vi "rs3_ReadDepthPreference3.vi"(0 "file (use dialog)":path) -> (1 "HDAD 2*":T1={"lambdaCensus"=126.0, "lambdaAD"=800.0, "ignoreSAD"=0}, 3 "ST Color Control 2":T4, 4 "depth control 2":T8={"plusIncrement (47)"=19, "MinusDecrement (46)"=4, "deepSeaMedianThreshold (48)"=554, "scoreThreshA(49)"=1, "scoreThreshB (50)"=632, "textureDifferenceThreshold (52)"=0, "textureCountThreshold (51)"=32, "deepSea2ndPeakThresh.(53)"=665, "deepSeaNeighborThresh.(54)"=126, "IrAgreeThreshold (55)"=11}, 6 "ST RSM 2":T7={"rsmBypass (56)"=0, "diffThresh (57)"=6.49, "sloRauDiffThresh(58)"=0.305, "removeThresh(59)"=60}, 9 "text":string="{\n    \"param-disableraucolor\": 0,\n    \"param-disablesadcolor\": 0,\n    \"param-disablesadnormalize\": 0,\n    \"param-disablesloleftcolor\": 0,\n    \"param-disableslorightcolor\": 0,\n    \"param-lambdaad\": 833,\n    \"param-lambdacensus\": 26,\n    \"param-leftrightthreshold\": 11,\n    \"param-maxscorethreshb\": 632,\n    \"param-medianthreshold\": 554,\n    \"param-minscorethresha\": 1,\n    \"param-neighborthresh\": 126,\n    \"param-raumine\": 7,\n    \"param-rauminn\": 1,\n    \"param-rauminnssum\": 7,\n    \"param-raumins\": 3,\n    \"param-rauminw\": 5,\n    \"param-rauminwesum\": 12,\n    \"param-regioncolorthresholdb\": 0.26379450841061053,\n    \"param-regioncolorthresholdg\": 0.9806201235330119,\n    \"param-regioncolorthresholdr\": 0.013826660558426103,\n    \"param-regionshrinku\": 4,\n    \"param-regionshrinkv\": 1,\n    \"param-regionspatialthresholdu\": 7,\n    \"param-regionspatialthresholdv\": 3,\n    \"param-robbinsmonrodecrement\": 4,\n    \"param-robbinsmonroincrement\": 19,\n    \"param-rsmdiffthreshold\": 1.0367311077984247,\n    \"param-rsmrauslodiffthreshold\": 0.8955340364089305,\n    \"param-rsmremovethreshold\": 0.7604262237190709,\n    \"param-scanlineedgetaub\": 105,\n    \"param-scanlineedgetaug\": 442,\n    \"param-scanlineedgetaur\": 46,\n    \"param-scanlinep1\": 93,\n    \"param-scanlinep1onediscon\": 70,\n    \"param-scanlinep1twodiscon\": 92,\n    \"param-scanlinep2\": 473,\n    \"param-scanlinep2onediscon\": 123,\n    \"param-scanlinep2twodiscon\": 409,\n    \"param-secondpeakdelta\": 665,\n    \"param-texturecountthresh\": 32,\n    \"param-texturedifferencethresh\": 0,\n    \"param-usersm\": 1\n}", 10 "ST SLO Penalty 2":T6={"sloK1Penalty (79)"=10, "sloK2Penalty (80)"=60, "sloK1PenaltyMod1(81)"=84, "sloK2PenaltyMod1(82)"=56, "sloK1PenaltyMod2(83)"=59, "sloK2PenaltyMod2(84)"=4}, 12 "ST SLO Threshold 2":T2={"SLOdiffThreshRed(76)"=200, "SLODiffThreshGreen(77)"=200, "SLODiffThreshBlue(78)"=200}, 13 "error out":errorcluster, 14 "ST Rau Threshold 2":T3={"rauDiffThreshRed(73)"=70, "rauDiffThreshGreen(74)"=70, "rauDiffThreshBlue(75)"=70}, 15 "ST RAU vector 2":T5={"minWest (60)"=7, "minEast (61)"=7, "minWEsum (62)"=12, "minNorth (63)"=3, "minSouth (64)"=2, "minNSSum(65)"=1, "uStrink (66)"=2, "vShrink (67)"=1})   [LabVIEW 2019, in "libRealSense3.lvlib"]
uses:
  libRealSense3.lvlib
panel:
  in  "error in (no error)":errorcluster
  # "RS2 Read Depth Preferences"
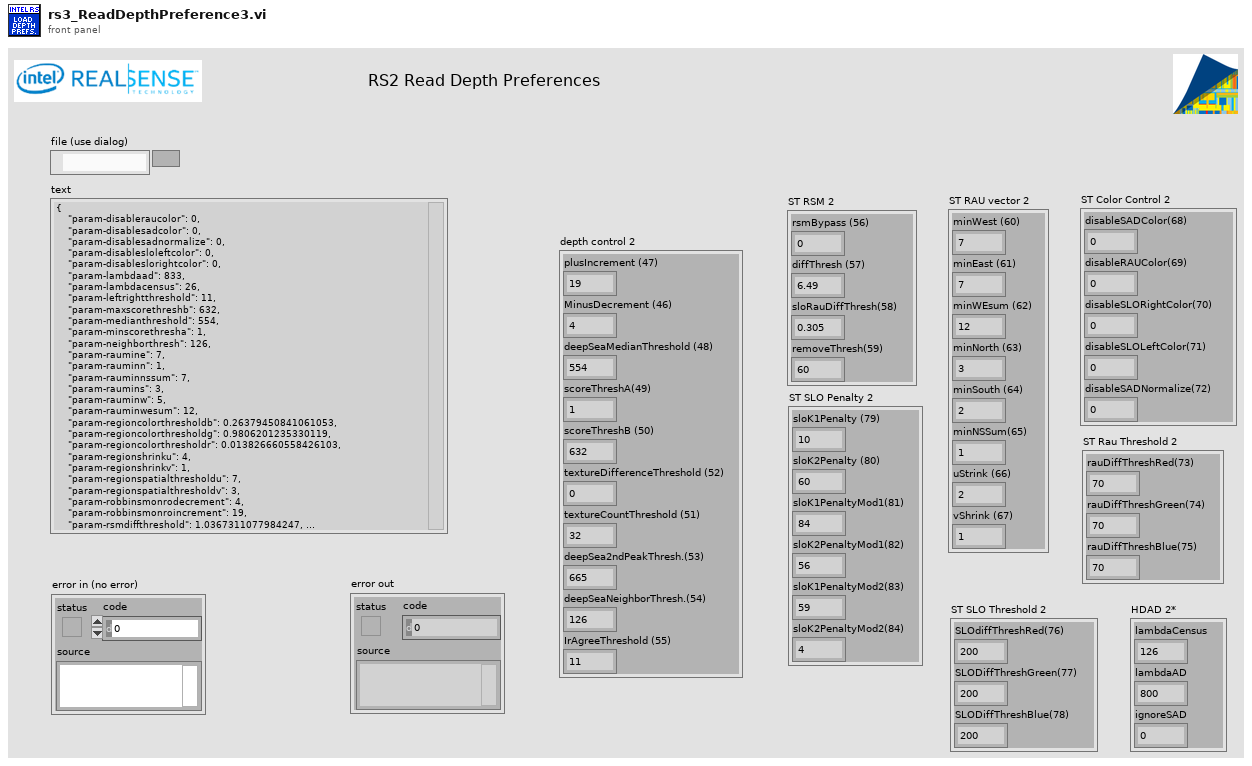
[diagram p1: front panel]
types:
  T1 = cluster{"lambdaCensus":sgl, "lambdaAD":sgl, "ignoreSAD":u32}
  T2 = cluster{"SLOdiffThreshRed(76)":u32, "SLODiffThreshGreen(77)":u32, "SLODiffThreshBlue(78)":u32}
  T3 = cluster{"rauDiffThreshRed(73)":u32, "rauDiffThreshGreen(74)":u32, "rauDiffThreshBlue(75)":u32}
  T4 = cluster{"disableSADColor(68)":u32, "disableRAUColor(69)":u32, "disableSLORightColor(70)":u32, "disableSLOLeftColor(71)":u32, "disableSADNormalize(72)":u32}
  T5 = cluster{"minWest (60)":u32, "minEast (61)":u32, "minWEsum (62)":u32, "minNorth (63)":u32, "minSouth (64)":u32, "minNSSum(65)":u32, "uStrink (66)":u32, "vShrink (67)":u32}
  T6 = cluster{"sloK1Penalty (79)":u32, "sloK2Penalty (80)":u32, "sloK1PenaltyMod1(81)":u32, "sloK2PenaltyMod1(82)":u32, "sloK1PenaltyMod2(83)":u32, "sloK2PenaltyMod2(84)":u32}
  T7 = cluster{"rsmBypass (56)":u32, "diffThresh (57)":sgl, "sloRauDiffThresh(58)":sgl, "removeThresh(59)":u32}
  T8 = cluster{"plusIncrement (47)":u32, "MinusDecrement (46)":u32, "deepSeaMedianThreshold (48)":u32, "scoreThreshA(49)":u32, "scoreThreshB (50)":u32, "textureDifferenceThreshold (52)":u32, "textureCountThreshold (51)":u32, "deepSea2ndPeakThresh.(53)":u32, "deepSeaNeighborThresh.(54)":u32, "IrAgreeThreshold (55)":u32}
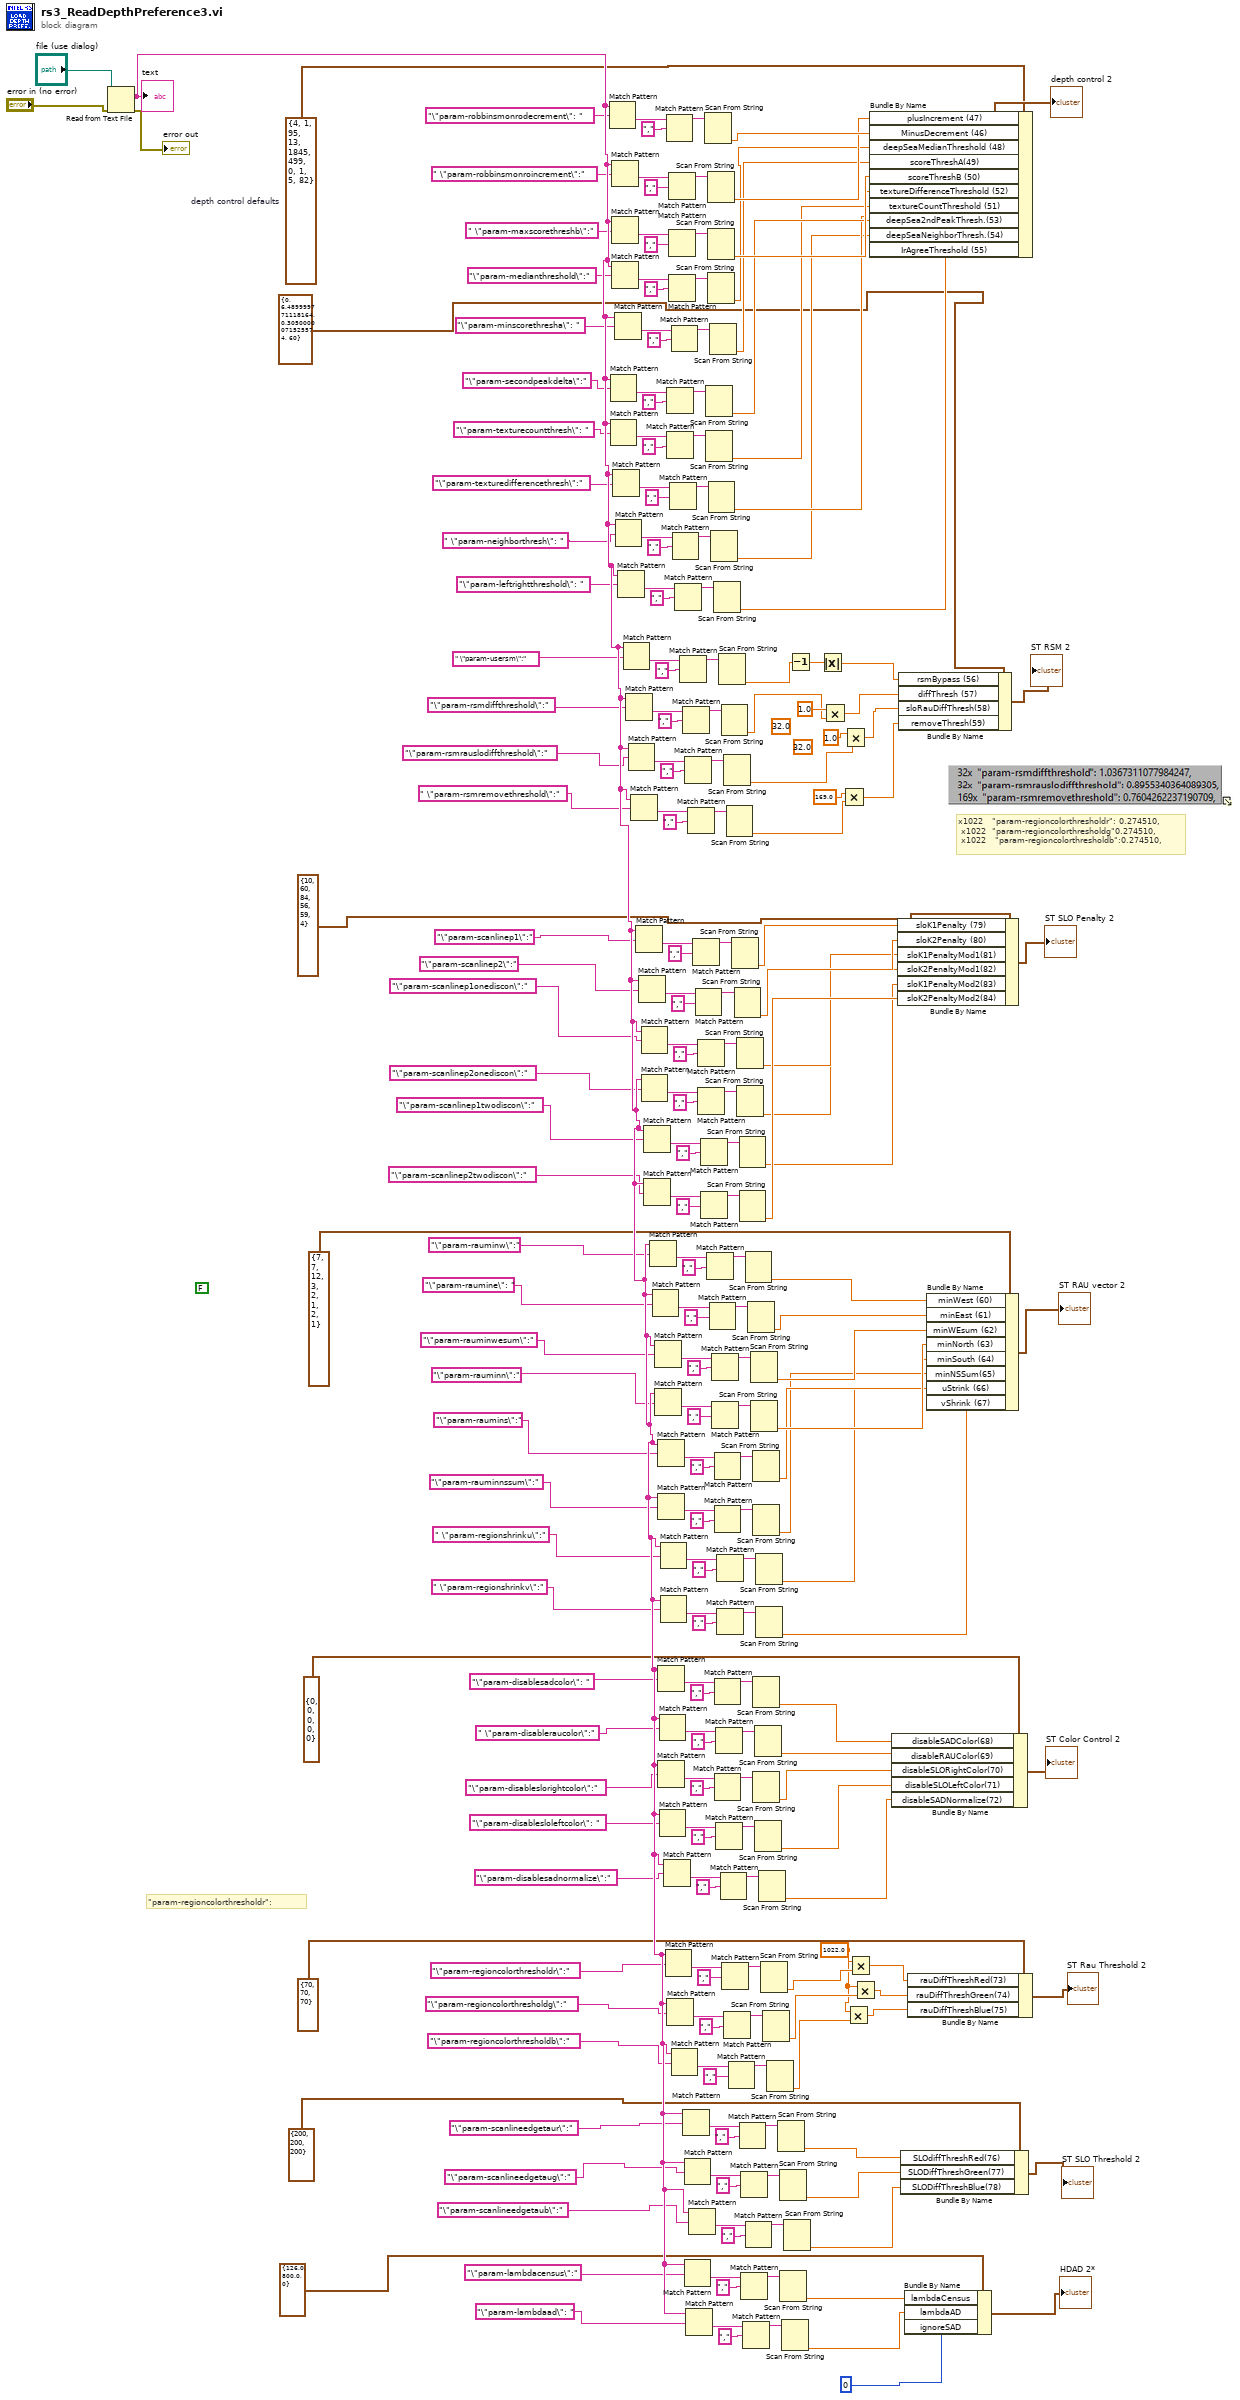
[diagram p0: block diagram]
diagram:
  (unwired) 32.0 ("x")
  (unwired) 32.0 ("x")
  w8 = 1022.0
  w229 = T8 {"plusIncrement (47)"=4, "MinusDecrement (46)"=1, "deepSeaMedianThreshold (48)"=95, "scoreThreshA(49)"=13, "scoreThreshB (50)"=1845, "textureDifferenceThreshold (52)"=499, "textureCountThreshold (51)"=0, "deepSea2ndPeakThresh.(53)"=1, "deepSeaNeighborThresh.(54)"=5, "IrAgreeThreshold (55)"=82}  # depth control defaults
  (unwired) FALSE
  # "x1022   \"param-regioncolorthresholdr\": 0.274510, \n x1022  \"param-regioncolorthresholdg\"0.274510, \n x1022   \"param-regioncolorthresholdb\":0.274510,"
  # "\"param-regioncolorthresholdr\":"
  n1 = Read from Text File(file (use dialog)="file (use dialog)", error in="error in (no error)") -> (text=w238:string, error out=→"error out":errorcluster)  [unwired: 2 in, 2 out]
  "text" <- w238
  n2 = Match Pattern(string=w238, regular expression="\"param-robbinsmonrodecrement\": ") -> (after substring=w235:string)  [unwired: 1 in, 3 out]
  n3 = Match Pattern(string=w238, regular expression="\"param-secondpeakdelta\":") -> (after substring=w203:string)  [unwired: 1 in, 3 out]
  n4 = Match Pattern(string=w238, regular expression="\"param-texturecountthresh\": ") -> (after substring=w208:string)  [unwired: 1 in, 3 out]
  n5 = Match Pattern(string=w238, regular expression=" \"param-robbinsmonroincrement\":") -> (after substring=w232:string)  [unwired: 1 in, 3 out]
  n6 = Match Pattern(string=w238, regular expression=" \"param-maxscorethreshb\":") -> (after substring=w224:string)  [unwired: 1 in, 3 out]
  n7 = Match Pattern(string=w238, regular expression="\"param-medianthreshold\":") -> (after substring=w219:string)  [unwired: 1 in, 3 out]
  n8 = Match Pattern(string=w238, regular expression="\"param-texturedifferencethresh\":") -> (after substring=w209:string)  [unwired: 1 in, 3 out]
  n9 = Match Pattern(string=w238, regular expression="\"param-minscorethresha\": ") -> (after substring=w218:string)  [unwired: 1 in, 3 out]
  n10 = Match Pattern(string=w238, regular expression=" \"param-neighborthresh\": ") -> (after substring=w194:string)  [unwired: 1 in, 3 out]
  n11 = Match Pattern(string=w238, regular expression="\"param-leftrightthreshold\": ") -> (after substring=w193:string)  [unwired: 1 in, 3 out]
  n12 = Match Pattern(string=w238, regular expression=" \"param-usersm\":") -> (after substring=w175:string)  [unwired: 1 in, 3 out]
  n13 = Match Pattern(string=w238, regular expression="\"param-rsmdiffthreshold\":") -> (after substring=w174:string)  [unwired: 1 in, 3 out]
  n14 = Match Pattern(string=w238, regular expression="\"param-rsmrauslodiffthreshold\":") -> (after substring=w180:string)  [unwired: 1 in, 3 out]
  n15 = Match Pattern(string=w238, regular expression=" \"param-rsmremovethreshold\":") -> (after substring=w181:string)  [unwired: 1 in, 3 out]
  n16 = Match Pattern(string=w238, regular expression="\"param-scanlinep1\":") -> (after substring=w162:string)  [unwired: 1 in, 3 out]
  n17 = Match Pattern(string=w238, regular expression="\"param-scanlinep2\":") -> (after substring=w159:string)  [unwired: 1 in, 3 out]
  n18 = Match Pattern(string=w238, regular expression="\"param-scanlinep1onediscon\":") -> (after substring=w158:string)  [unwired: 1 in, 3 out]
  n19 = Match Pattern(string=w238, regular expression="\"param-scanlinep2onediscon\":") -> (after substring=w153:string)  [unwired: 1 in, 3 out]
  n20 = Match Pattern(string=w238, regular expression="\"param-scanlinep1twodiscon\":") -> (after substring=w152:string)  [unwired: 1 in, 3 out]
  n21 = Match Pattern(string=w238, regular expression="\"param-scanlinep2twodiscon\":") -> (after substring=w143:string)  [unwired: 1 in, 3 out]
  n22 = Match Pattern(string=w238, regular expression="\"param-rauminw\":") -> (after substring=w115:string)  [unwired: 1 in, 3 out]
  n23 = Match Pattern(string=w238, regular expression="\"param-raumine\": ") -> (after substring=w118:string)  [unwired: 1 in, 3 out]
  n24 = Match Pattern(string=w238, regular expression="\"param-rauminwesum\":") -> (after substring=w119:string)  [unwired: 1 in, 3 out]
  n25 = Match Pattern(string=w238, regular expression="\"param-rauminn\":") -> (after substring=w124:string)  [unwired: 1 in, 3 out]
  n26 = Match Pattern(string=w238, regular expression="\"param-raumins\":") -> (after substring=w125:string)  [unwired: 1 in, 3 out]
  n27 = Match Pattern(string=w238, regular expression="\"param-rauminnssum\":") -> (after substring=w130:string)  [unwired: 1 in, 3 out]
  n28 = Match Pattern(string=w238, regular expression="\"param-disablesadcolor\": ") -> (after substring=w88:string)  [unwired: 1 in, 3 out]
  n29 = Match Pattern(string=w238, regular expression="\"param-disableslorightcolor\":") -> (after substring=w77:string)  [unwired: 1 in, 3 out]
  n30 = Match Pattern(string=w238, regular expression=" \"param-disableraucolor\":") -> (after substring=w83:string)  [unwired: 1 in, 3 out]
  n31 = Match Pattern(string=w238, regular expression="\"param-disablesloleftcolor\": ") -> (after substring=w82:string)  [unwired: 1 in, 3 out]
  n32 = Match Pattern(string=w238, regular expression=" \"param-regionshrinku\":") -> (after substring=w112:string)  [unwired: 1 in, 3 out]
  n33 = Match Pattern(string=w238, regular expression=" \"param-regionshrinkv\":") -> (after substring=w107:string)  [unwired: 1 in, 3 out]
  n34 = Match Pattern(string=w238, regular expression="\"param-disablesadnormalize\":") -> (after substring=w74:string)  [unwired: 1 in, 3 out]
  n35 = Match Pattern(string=w238, regular expression="\"param-regioncolorthresholdr\":") -> (after substring=w59:string)  [unwired: 1 in, 3 out]
  n36 = Match Pattern(string=w235, regular expression=",") -> (before substring=w237:string)  [unwired: 1 in, 3 out]
  n37 = Match Pattern(string=w203, regular expression=",") -> (before substring=w205:string)  [unwired: 1 in, 3 out]
  n38 = Match Pattern(string=w208, regular expression=",") -> (before substring=w206:string)  [unwired: 1 in, 3 out]
  n39 = Match Pattern(string=w238, regular expression="\"param-regioncolorthresholdg\":") -> (after substring=w54:string)  [unwired: 1 in, 3 out]
  n40 = Match Pattern(string=w232, regular expression=",") -> (before substring=w231:string)  [unwired: 1 in, 3 out]
  n41 = Match Pattern(string=w224, regular expression=",") -> (before substring=w222:string)  [unwired: 1 in, 3 out]
  n42 = Match Pattern(string=w219, regular expression=",") -> (before substring=w221:string)  [unwired: 1 in, 3 out]
  n43 = Match Pattern(string=w209, regular expression=",") -> (before substring=w211:string)  [unwired: 1 in, 3 out]
  n44 = Match Pattern(string=w218, regular expression=",") -> (before substring=w216:string)  [unwired: 1 in, 3 out]
  n45 = Match Pattern(string=w238, regular expression="\"param-regioncolorthresholdb\":") -> (after substring=w62:string)  [unwired: 1 in, 3 out]
  n46 = Match Pattern(string=w194, regular expression=",") -> (before substring=w196:string)  [unwired: 1 in, 3 out]
  n47 = Match Pattern(string=w193, regular expression=",") -> (before substring=w191:string)  [unwired: 1 in, 3 out]
  n48 = Match Pattern(string=w175, regular expression=",") -> (before substring=w177:string)  [unwired: 1 in, 3 out]
  n49 = Match Pattern(string=w174, regular expression=",") -> (before substring=w172:string)  [unwired: 1 in, 3 out]
  n50 = Match Pattern(string=w238, regular expression="\"param-scanlineedgetaur\":") -> (after substring=w45:string)  [unwired: 1 in, 3 out]
  n51 = Match Pattern(string=w238, regular expression="\"param-scanlineedgetaug\":") -> (after substring=w50:string)  [unwired: 1 in, 3 out]
  n52 = Match Pattern(string=w238, regular expression="\"param-lambdacensus\":") -> (after substring=w38:string)  [unwired: 1 in, 3 out]
  n53 = Match Pattern(string=w180, regular expression=",") -> (before substring=w178:string)  [unwired: 1 in, 3 out]
  n54 = Match Pattern(string=w238, regular expression="\"param-lambdaad\": ") -> (after substring=w33:string)  [unwired: 1 in, 3 out]
  n55 = Match Pattern(string=w181, regular expression=",") -> (before substring=w183:string)  [unwired: 1 in, 3 out]
  n56 = Match Pattern(string=w238, regular expression="\"param-scanlineedgetaub\":") -> (after substring=w42:string)  [unwired: 1 in, 3 out]
  n57 = Match Pattern(string=w162, regular expression=",") -> (before substring=w164:string)  [unwired: 1 in, 3 out]
  n58 = Match Pattern(string=w159, regular expression=",") -> (before substring=w161:string)  [unwired: 1 in, 3 out]
  n59 = Match Pattern(string=w158, regular expression=",") -> (before substring=w156:string)  [unwired: 1 in, 3 out]
  n60 = Match Pattern(string=w153, regular expression=",") -> (before substring=w155:string)  [unwired: 1 in, 3 out]
  n61 = Match Pattern(string=w152, regular expression=",") -> (before substring=w150:string)  [unwired: 1 in, 3 out]
  n62 = Match Pattern(string=w143, regular expression=",") -> (before substring=w145:string)  [unwired: 1 in, 3 out]
  n63 = Scan From String(input string=w237) -> (output 1=w228:dbl)  [unwired: 4 in, 3 out]
  n64 = Scan From String(input string=w205) -> (output 1=w199:dbl)  [unwired: 4 in, 3 out]
  n65 = Scan From String(input string=w206) -> (output 1=w198:dbl)  [unwired: 4 in, 3 out]
  n66 = Match Pattern(string=w115, regular expression=",") -> (before substring=w113:string)  [unwired: 1 in, 3 out]
  n67 = Scan From String(input string=w231) -> (output 1=w227:dbl)  [unwired: 4 in, 3 out]
  n68 = Scan From String(input string=w222) -> (output 1=w214:dbl)  [unwired: 4 in, 3 out]
  n69 = Scan From String(input string=w221) -> (output 1=w212:dbl)  [unwired: 4 in, 3 out]
  n70 = Scan From String(input string=w211) -> (output 1=w197:dbl)  [unwired: 4 in, 3 out]
  n71 = Match Pattern(string=w118, regular expression=",") -> (before substring=w116:string)  [unwired: 1 in, 3 out]
  n72 = Scan From String(input string=w216) -> (output 1=w213:dbl)  [unwired: 4 in, 3 out]
  n73 = Scan From String(input string=w196) -> (output 1=w189:dbl)  [unwired: 4 in, 3 out]
  n74 = Match Pattern(string=w119, regular expression=",") -> (before substring=w121:string)  [unwired: 1 in, 3 out]
  n75 = Match Pattern(string=w124, regular expression=",") -> (before substring=w122:string)  [unwired: 1 in, 3 out]
  n76 = Scan From String(input string=w191) -> (output 1=w186:dbl)  [unwired: 4 in, 3 out]
  n77 = Match Pattern(string=w125, regular expression=",") -> (before substring=w127:string)  [unwired: 1 in, 3 out]
  n78 = Match Pattern(string=w130, regular expression=",") -> (before substring=w128:string)  [unwired: 1 in, 3 out]
  n79 = Match Pattern(string=w88, regular expression=",") -> (before substring=w86:string)  [unwired: 1 in, 3 out]
  n80 = Match Pattern(string=w77, regular expression=",") -> (before substring=w79:string)  [unwired: 1 in, 3 out]
  n81 = Match Pattern(string=w83, regular expression=",") -> (before substring=w85:string)  [unwired: 1 in, 3 out]
  n82 = Match Pattern(string=w82, regular expression=",") -> (before substring=w80:string)  [unwired: 1 in, 3 out]
  n83 = Match Pattern(string=w112, regular expression=",") -> (before substring=w110:string)  [unwired: 1 in, 3 out]
  n84 = Match Pattern(string=w107, regular expression=",") -> (before substring=w109:string)  [unwired: 1 in, 3 out]
  n85 = Scan From String(input string=w177) -> (output 1=w165:dbl)  [unwired: 4 in, 3 out]
  n86 = Match Pattern(string=w74, regular expression=",") -> (before substring=w76:string)  [unwired: 1 in, 3 out]
  n87 = Scan From String(input string=w172) -> (output 1=w6:dbl)  [unwired: 4 in, 3 out]
  n88 = Match Pattern(string=w59, regular expression=",") -> (before substring=w57:string)  [unwired: 1 in, 3 out]
  n89 = Scan From String(input string=w178) -> (output 1=w25:dbl)  [unwired: 4 in, 3 out]
  n90 = Match Pattern(string=w54, regular expression=",") -> (before substring=w56:string)  [unwired: 1 in, 3 out]
  n91 = Scan From String(input string=w183) -> (output 1=w3:dbl)  [unwired: 4 in, 3 out]
  n92 = Match Pattern(string=w62, regular expression=",") -> (before substring=w60:string)  [unwired: 1 in, 3 out]
  n93 = Scan From String(input string=w164) -> (output 1=w140:dbl)  [unwired: 4 in, 3 out]
  n94 = Scan From String(input string=w161) -> (output 1=w139:dbl)  [unwired: 4 in, 3 out]
  n95 = Scan From String(input string=w156) -> (output 1=w138:dbl)  [unwired: 4 in, 3 out]
  n96 = Scan From String(input string=w155) -> (output 1=w134:dbl)  [unwired: 4 in, 3 out]
  n97 = Scan From String(input string=w150) -> (output 1=w133:dbl)  [unwired: 4 in, 3 out]
  n98 = Scan From String(input string=w145) -> (output 1=w141:dbl)  [unwired: 4 in, 3 out]
  n99 = Match Pattern(string=w45, regular expression=",") -> (before substring=w47:string)  [unwired: 1 in, 3 out]
  n100 = Match Pattern(string=w50, regular expression=",") -> (before substring=w48:string)  [unwired: 1 in, 3 out]
  n101 = Match Pattern(string=w38, regular expression=",") -> (before substring=w36:string)  [unwired: 1 in, 3 out]
  n102 = Match Pattern(string=w33, regular expression=",") -> (before substring=w35:string)  [unwired: 1 in, 3 out]
  n103 = Scan From String(input string=w113) -> (output 1=w106:dbl)  [unwired: 4 in, 3 out]
  n104 = Match Pattern(string=w42, regular expression=",") -> (before substring=w44:string)  [unwired: 1 in, 3 out]
  n105 = Scan From String(input string=w116) -> (output 1=w105:dbl)  [unwired: 4 in, 3 out]
  n106 = Scan From String(input string=w121) -> (output 1=w104:dbl)  [unwired: 4 in, 3 out]
  n107 = Scan From String(input string=w122) -> (output 1=w103:dbl)  [unwired: 4 in, 3 out]
  n108 = Scan From String(input string=w127) -> (output 1=w102:dbl)  [unwired: 4 in, 3 out]
  n109 = Scan From String(input string=w128) -> (output 1=w101:dbl)  [unwired: 4 in, 3 out]
  n110 = Scan From String(input string=w86) -> (output 1=w73:dbl)  [unwired: 4 in, 3 out]
  n111 = Scan From String(input string=w79) -> (output 1=w71:dbl)  [unwired: 4 in, 3 out]
  n112 = Scan From String(input string=w85) -> (output 1=w72:dbl)  [unwired: 4 in, 3 out]
  n113 = Scan From String(input string=w80) -> (output 1=w70:dbl)  [unwired: 4 in, 3 out]
  n114 = Scan From String(input string=w110) -> (output 1=w100:dbl)  [unwired: 4 in, 3 out]
  n115 = Scan From String(input string=w109) -> (output 1=w99:dbl)  [unwired: 4 in, 3 out]
  n116 = Scan From String(input string=w76) -> (output 1=w69:dbl)  [unwired: 4 in, 3 out]
  n117 = Scan From String(input string=w57) -> (output 1=w14:dbl)  [unwired: 4 in, 3 out]
  n118 = Scan From String(input string=w56) -> (output 1=w12:dbl)  [unwired: 4 in, 3 out]
  n119 = Scan From String(input string=w60) -> (output 1=w9:dbl)  [unwired: 4 in, 3 out]
  n120 = Scan From String(input string=w47) -> (output 1=w41:dbl)  [unwired: 4 in, 3 out]
  n121 = Scan From String(input string=w48) -> (output 1=w40:dbl)  [unwired: 4 in, 3 out]
  n122 = Scan From String(input string=w36) -> (output 1=w28:dbl)  [unwired: 4 in, 3 out]
  n123 = Scan From String(input string=w35) -> (output 1=w27:dbl)  [unwired: 4 in, 3 out]
  n124 = Scan From String(input string=w44) -> (output 1=w39:dbl)  [unwired: 4 in, 3 out]
  n125 = Decrement(x=w165) -> (x-1=w166:dbl)
  n126 = Absolute Value(x=w166) -> (abs(x)=w167:dbl)
  n127 = Multiply(x=1.0, y=w6) -> (x*y=w5:dbl)
  n128 = Multiply(x=169.0, y=w3) -> (x*y=w2:dbl)
  n129 = Multiply(x=1.0, y=w25) -> (x*y=w23:dbl)
  n130 = Multiply(x=w8, y=w9) -> (x*y=w10:dbl)
  n131 = Multiply(x=w8, y=w14) -> (x*y=w13:dbl)
  n132 = Multiply(x=w8, y=w12) -> (x*y=w11:dbl)
  n133 = Bundle By Name(cluster=w229, "plusIncrement (47)"=w227, "MinusDecrement (46)"=w228, "deepSeaMedianThreshold (48)"=w212, "scoreThreshA(49)"=w213, "scoreThreshB (50)"=w214, "textureDifferenceThreshold (52)"=w197, "textureCountThreshold (51)"=w198, "deepSea2ndPeakThresh.(53)"=w199, "deepSeaNeighborThresh.(54)"=w189, "IrAgreeThreshold (55)"=w186) -> (→"depth control 2":T8)
  n134 = Bundle By Name(cluster=T4 {"disableSADColor(68)"=0, "disableRAUColor(69)"=0, "disableSLORightColor(70)"=0, "disableSLOLeftColor(71)"=0, "disableSADNormalize(72)"=0} ("ST Color Control 2"), "disableSADColor(68)"=w73, "disableRAUColor(69)"=w72, "disableSLORightColor(70)"=w71, "disableSLOLeftColor(71)"=w70, "disableSADNormalize(72)"=w69) -> (→"ST Color Control 2":T4)
  n135 = Bundle By Name(cluster=T6 {"sloK1Penalty (79)"=10, "sloK2Penalty (80)"=60, "sloK1PenaltyMod1(81)"=84, "sloK2PenaltyMod1(82)"=56, "sloK1PenaltyMod2(83)"=59, "sloK2PenaltyMod2(84)"=4} ("ST SLO Penalty 2"), "sloK1Penalty (79)"=w140, "sloK2Penalty (80)"=w139, "sloK1PenaltyMod1(81)"=w138, "sloK2PenaltyMod1(82)"=w134, "sloK1PenaltyMod2(83)"=w133, "sloK2PenaltyMod2(84)"=w141) -> (→"ST SLO Penalty 2":T6)
  n136 = Bundle By Name(cluster=T7 {"rsmBypass (56)"=0, "diffThresh (57)"=6.49, "sloRauDiffThresh(58)"=0.305, "removeThresh(59)"=60} ("ST RSM 2"), "rsmBypass (56)"=w167, "diffThresh (57)"=w5, "sloRauDiffThresh(58)"=w23, "removeThresh(59)"=w2) -> (→"ST RSM 2":T7)
  n137 = Bundle By Name(cluster=T2 {"SLOdiffThreshRed(76)"=200, "SLODiffThreshGreen(77)"=200, "SLODiffThreshBlue(78)"=200} ("ST SLO Threshold 2"), "SLOdiffThreshRed(76)"=w41, "SLODiffThreshGreen(77)"=w40, "SLODiffThreshBlue(78)"=w39) -> (→"ST SLO Threshold 2":T2)
  n138 = Bundle By Name(cluster=T1 {"lambdaCensus"=126.0, "lambdaAD"=800.0, "ignoreSAD"=0} ("HDAD 2*"), "lambdaCensus"=w28, "lambdaAD"=w27, "ignoreSAD"=u32 0) -> (→"HDAD 2*":T1)
  n139 = Bundle By Name(cluster=T3 {"rauDiffThreshRed(73)"=70, "rauDiffThreshGreen(74)"=70, "rauDiffThreshBlue(75)"=70} ("ST Rau Threshold 2"), "rauDiffThreshRed(73)"=w13, "rauDiffThreshGreen(74)"=w11, "rauDiffThreshBlue(75)"=w10) -> (→"ST Rau Threshold 2":T3)
  n140 = Bundle By Name(cluster=T5 {"minWest (60)"=7, "minEast (61)"=7, "minWEsum (62)"=12, "minNorth (63)"=3, "minSouth (64)"=2, "minNSSum(65)"=1, "uStrink (66)"=2, "vShrink (67)"=1} ("ST RAU vector 2"), "minWest (60)"=w106, "minEast (61)"=w105, "minWEsum (62)"=w104, "minNorth (63)"=w103, "minSouth (64)"=w102, "minNSSum(65)"=w101, "uStrink (66)"=w100, "vShrink (67)"=w99) -> (→"ST RAU vector 2":T5)
